vi "Read pattern.vi"(8 "error in (no error)":errorcluster, 11 "TreeDirectoryExt in":refnum<class "TreeDirectoryExt.lvclass">) -> (0 "error out":errorcluster, 2 "pattern":string, 3 "TreeDirectoryExt out":refnum<class "TreeDirectoryExt.lvclass">)   [LabVIEW 2026, in "TreeDirectoryExt.lvclass"]
uses:
  TreeDirectoryExt.lvclass
  TreeDirectoryExt.lvclass/TreeDirectoryExt.ctl
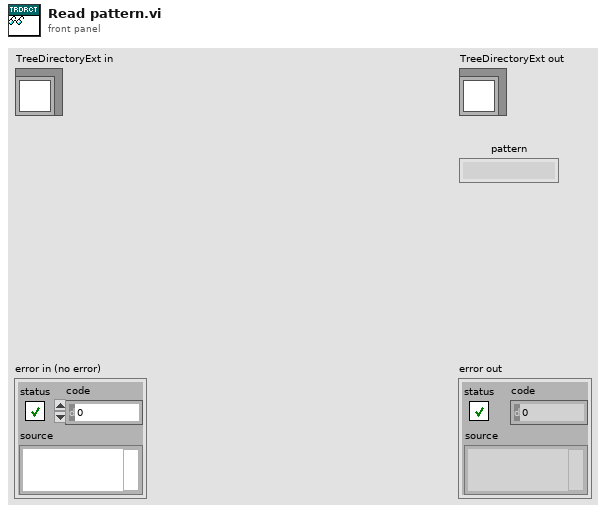
[diagram p1: front panel]
types:
  T1 = typedef "TreeDirectoryExt.lvclass/State Data.ctl" = cluster{"IconLibrary":variant, "pattern":string, "Clear Tree on Exit?":bool}
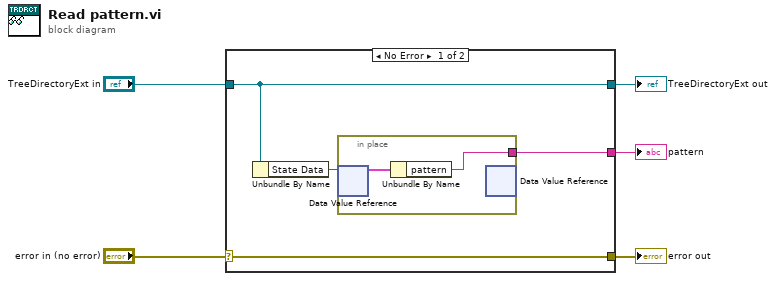
[diagram p0: block diagram]
diagram:
  n1 = case shown="No Error" "error in (no error)" {
    selector: "error in (no error)" -> [w9 w12]
    tunnel: [w9 w12] -> w4
    tunnel: [w8 w13] -> w2
    tunnel: "TreeDirectoryExt in" -> [w8 w13]
    tunnel: [w6 _] -> w1
    frame No Error {
      n2 = Unbundle By Name(w8) -> ("State Data"=w7:refnum<data-value>)
      n3 = in-place {
        in-place-border: [w10] -> w6
        n4 = in-place-dvr #1(w7) -> (w11:T1)  [unwired: 1 out]
        n5 = Unbundle By Name(w11) -> ("pattern"=w10:string)
        n6 = in-place-dvr #1() -> ()  [unwired: 1 in, 2 out]
      }
    }
    frame Error {
    }
  }
  "error out" <- w4
  "TreeDirectoryExt out" <- w2
  "pattern" <- w1
